vi "GPS Waypoint List Recorder FPGA.vi"(10 "Read Point?":bool) -> ()   [LabVIEW 2009]
uses:
  <vilib>/rvi/interface/nirviOpenFPGA/nirviOpenFPGA.xnode
  FPGA Bitfiles/Q_IGVC_2010.lvproj_FPGA Target_FPGA_MAIN.vi.lvbitx
  <vilib>/userDefined/High Color/nirio_resource_hc.ctl
  <vilib>/LabVIEW Targets/FPGA/cRIO/shared/nicrio_ModuleControls/nicrio_cRIO-9871_DataBitsEnum.ctl
  <vilib>/LabVIEW Targets/FPGA/cRIO/shared/nicrio_ModuleControls/nicrio_cRIO-9871_FlowControlEnum.ctl
  <vilib>/LabVIEW Targets/FPGA/cRIO/shared/nicrio_ModuleControls/nicrio_cRIO-9871_BaudRateEnum.ctl
  <vilib>/LabVIEW Targets/FPGA/cRIO/shared/nicrio_ModuleControls/nicrio_cRIO-9871_ParityEnum.ctl
  <vilib>/LabVIEW Targets/FPGA/cRIO/shared/nicrio_ModuleControls/nicrio_cRIO-9871_StopBitsEnum.ctl
  <vilib>/rvi/interface/nirviMethod/nirviMethod.xnode
  <vilib>/rvi/interface/common/niFpgaNodeNameForErrorReporting.ctl
  <vilib>/rvi/errors/niLvFpgaWhatHappensToTopLevelVI.ctl
  <vilib>/rvi/errors/niLvFpgaAdjustHostInterfaceError.vi
  NiRioSrv.dll
  <vilib>/Utility/error.llb/Error Cluster From Error Code.vi
  <vilib>/rvi/interface/nirviCloseFPGA/nirviCloseFPGA.xnode
  TypeDefs/Sensor Typedefs/FPGA Main ref.ctl
  <vilib>/FPGAPlugInAG/cRIO-9113/nirviIntfOpen_cRIO-9113.vi
  <vilib>/Utility/error.llb/Merge Errors.vi
  <vilib>/LabVIEW Targets/FPGA/RIO/nirio_HostInterface/nirio_Reset.vi
  <vilib>/LabVIEW Targets/FPGA/RIO/nirio_HostInterface/nirio_DMAStopAll.vi
  <vilib>/LabVIEW Targets/FPGA/RIO/nirio_HostInterface/nirio_DisableInterrupts.vi
  <vilib>/RVI Host/nirviSupport.llb/nirviErrorClusterFromErrorCode.vi
  <vilib>/LabVIEW Targets/FPGA/RIO/nirio_HostInterface/nirio_EnableInterrupts.vi
  <vilib>/rvi/errors/niLvFpgaReportInternalErrorWithAdditionalInfo.vi
  <vilib>/FPGAPlugInAG/cRIO-9113/nirviIntfClose_cRIO-9113.vi
panel:
  in  "stop":bool
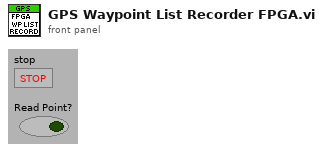
[diagram p1: front panel]
types:
  T1 = typedef "nicrio_cRIO-9871_StopBitsEnum.ctl" = enum8{"1", "1.5", "2"}
  T2 = typedef "nicrio_cRIO-9871_ParityEnum.ctl" = enum8{"None", "Odd", "Even", "Mark", "Space"}
  T3 = typedef "nicrio_cRIO-9871_BaudRateEnum.ctl" = enum16{"75 bps", "110 bps", "134 bps", "150 bps", "300 bps", "600 bps", "1200 bps", "1800 bps", "2400 bps", "4800 bps", "7200 bps", "9600 bps", "14.4 kbps", "19.2 kbps", "28.8 kbps", "38.4 kbps", "57.6 kbps", "115.2 kbps", "230.4 kbps", "460.8 kbps", "921.6 kbps"}
  T4 = typedef "nicrio_cRIO-9871_FlowControlEnum.ctl" = enum8{"None", "Software (XON / XOFF)", "Hardware (RTS / CTS)"}
  T5 = typedef "nicrio_cRIO-9871_DataBitsEnum.ctl" = enum8{"5", "6", "7", "8"}
  T6 = typedef "nirio_resource_hc.ctl" = tag
  T7 = enum16{"open", "replace", "create", "open or create", "replace or create", "replace or create with confirmation"}
  T8 = typedef "FPGA Main ref.ctl" = refnum<k20>
  T9 = typedef "EVS GPS Data.ctl" = cluster{"Latitude":dbl, "Longitude":dbl}
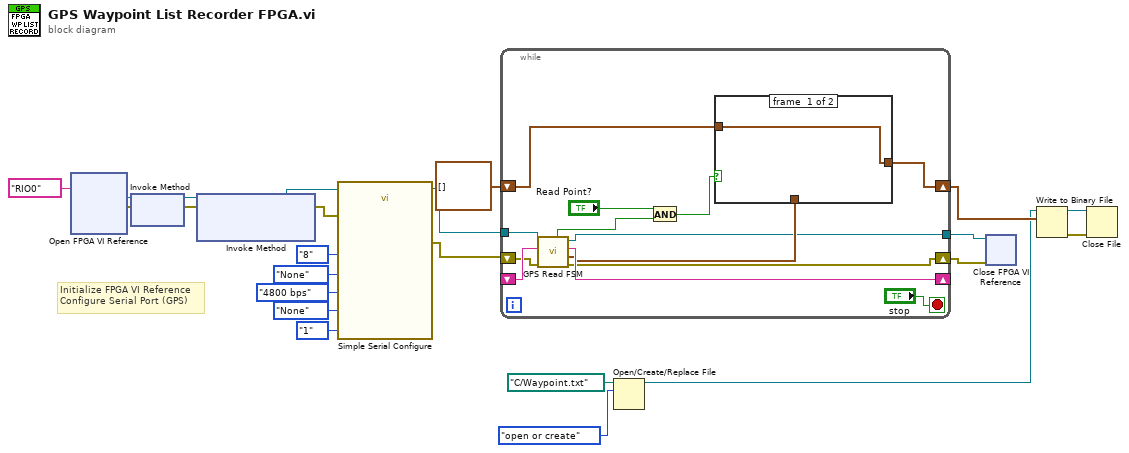
[diagram p0: block diagram]
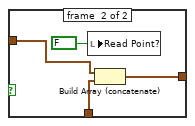
[diagram p2: hidden frame]
diagram:
  # "Initialize FPGA VI Reference\nConfigure Serial Port (GPS)"
  n1 = xnode "Open FPGA VI Reference"("resource name"=T6 "RIO0") -> ("FPGA VI Reference Out"=w10:refnum<k20>, "error out"=w9:errorcluster)  [unwired: 1 in]
  n2 = xnode "Invoke Method"("FPGA VI Reference In"=w10, "error in"=w9) -> ("FPGA VI Reference Out"=w8:refnum<k20>, "error out"=w7:errorcluster)
  n3 = xnode "Invoke Method"("FPGA VI Reference In"=w8, "error in"=w7) -> ("FPGA VI Reference Out"=w6:refnum<k20>, "error out"=w5:errorcluster)  [unwired: 1 in]
  n4 = call "Simple Serial Configure.vi"("Parity"=nicrio_cRIO-9871_ParityEnum."None", "Stop Bits"=nicrio_cRIO-9871_StopBitsEnum."1", "Flow Control"=nicrio_cRIO-9871_FlowControlEnum."None", "error in"=w5, "Data Bits"=nicrio_cRIO-9871_DataBitsEnum."8", "Baud Rate"=nicrio_cRIO-9871_BaudRateEnum."4800 bps", "FPGA VI Reference in"=w6) -> ("error out"=w3:errorcluster, "FPGA VI Reference out"=w4:T8)  [unwired: 3 in]
  n5 = while {
    shift-right: [w30] -> _
    shift-left: _ -> [w31]
    shift-right: [w28] -> w1
    shift-left: w3 -> [w29]
    shift-right: [w33] -> w21
    shift-left: cluster{"Longitude":dbl, "Latitude":dbl}[] [] -> [w34]
    tunnel: w4 -> [w32]
    tunnel: [w26] -> w2
    stop <- "stop" stop-if-true
    n6 = call "GPS Read FSM.vi"("error in (no error)"=w29, "header buffer in"=w31, "FPGA VI Reference in"=w32) -> ("error out"=w28:errorcluster, "GPS Buffer out"=w27:T9, "header buffer out"=w30:string, "FPGA VI Reference out"=w26:T8, "buffer updated"=w24:bool)  [unwired: 4 in]
    n7 = And(x="Read Point?", y=w24) -> (x .and. y?=w35:bool)
    n8 = case shown="True" w35 {
      tunnel: w34 -> [w37 w41]
      tunnel: [w37 w40] -> w33
      tunnel: w27 -> [_ w38]
      frame #0 {
      }
      frame #1 {
        n9 = local write "Read Point?"(FALSE ("Read Point?")) -> ()
        n10 = Build Array (concatenate)(w41, w38) -> (w40:T9[])
      }
    }
  }
  n11 = Open/Create/Replace File(file path (use dialog)=path "C:/Waypoint.txt", operation (0:open)=T7."open or create") -> (refnum out=w20:refnum<file>)  [unwired: 4 in, 2 out]
  n12 = xnode "Close FPGA VI Reference"("FPGA VI Reference In"=w2, "error in"=w1) -> ()  [unwired: 1 out]
  n13 = Write to Binary File(file (use dialog)=w20, data=w21) -> (refnum out=w19:refnum<file>, error out=w18:errorcluster)  [unwired: 4 in, 1 out]
  n14 = Close File(refnum=w19, error in=w18) -> ()  [unwired: 2 out]
